vi "AR_Online_Guide.vi"   [LabVIEW 2012]
uses:
  SubVIs/LVPresent_Globals.vi
panel:
  # "Get to know the board\n\nThe Arduino Uno is a relatively simple board to use, but you will need to wire it to a breadboard and various \n\nother elements to complete this tutorial. Whenever you see the                   image, you can find how to construct the circuit you need by clicking it.\n\n\nAlso, for the next two examples you will need pin 13, which is located here on the board."
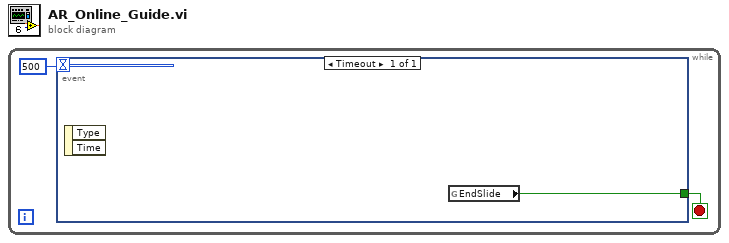
[diagram p0: block diagram]
diagram:
  n1 = while {
    stop <- w2 stop-if-true
    n2 = event shown="[0] Timeout" {
      selector: _ -> [_]
      dyn-events: _ -> [_]
      timeout: 500 -> [_]
      tunnel: [w3] -> w2
      event Timeout {
        n3 = event-data() -> ()  [unwired: 1 in, 2 out]
        n4 = global read "LVPresent_Globals.vi" "EndSlide"() -> (w3:bool)
      }
    }
  }
